vi "Actor Core.vi"(8 "error in":errorcluster, 11 "SensorViewDetailed in":refnum<class "TimerViewDetail.lvclass">) -> (0 "error out":errorcluster, 3 "Actor out":refnum<class "Actor.lvclass">)   [LabVIEW 2012, in "TimerSensor.lvlib" / "TimerViewDetail.lvclass"]
doc: "(<B>Filename</B>: Actor Framework.lvlib:Actor.lvclass:Actor Core.vi)\n\nReceives messages to the actor, reacts to them, and initiates any error handling that may shut the actor down.\n\nDescendant classes may override this VI to append parallel tasks for the actor to complete while it handles messages. Overrides use the Call Parent Method node."
uses:
  TimerViewDetail.lvclass
  <vilib>/ActorFramework/Actor/Actor.lvclass
  Sensor Definition/SensorViewDetailed.lvclass
  <vilib>/ActorFramework/Actor/Actor.lvclass/Actor.ctl
  <vilib>/ActorFramework/Message Enqueuer/Message Enqueuer.lvclass/Message Enqueuer.ctl
  Win8uiFramework/ViewableActor.lvclass/ViewableActor.ctl
  Sensor Definition/SensorView.lvclass/SensorView.ctl
  Sensor Messages/Request Detach Msg/Request Detach Msg.lvclass/Request Detach Msg.ctl
  TimerSensorConfig.lvclass
  Sensor Definition/SensorInfo.lvclass/SensorInfo.ctl
  TimerSensorConfig.lvclass/TimerSensorConfig.ctl
  Sensor Definition/Double Scalar SensorData.lvclass
  Sensor Definition/SensorInfo/Read Description.vi
  Sensor Definition/SensorInfo/Read Name.vi
  Sensor Definition/Read Config.vi
  TimerSensorConfig/Read Target Time.vi
  TimerSensorConfig/Read Timer Direction.vi
  Win8uiFramework/Read Stop Event.vi
  Sensor Definition/SensorView/Read SensorInfo Changed Event.vi
  Sensor Definition/SensorView/Read SensorData Changed Event.vi
  <vilib>/ActorFramework/Message Enqueuer/Init from Existing Queue.vi
  <vilib>/ActorFramework/Message Enqueuer/Enqueue.vi
  <vilib>/ActorFramework/Message Priority Queue/Priority Enqueue.vi
  <vilib>/ActorFramework/Message Enqueuer/Message Enqueuer.lvclass
  Sensor Definition/SensorInfo.lvclass
  Sensor Definition/SensorData.lvclass
  <vilib>/ActorFramework/Stop Msg/Stop Msg.lvclass
  Sensor Messages/Request Display Charm Msg/Request Display Charm Msg.lvclass
  Sensor Messages/Request Detach Msg/Request Detach Msg.lvclass
  Sensor Messages/Shutdown Sensor Msg/Shutdown Sensor Msg.lvclass
  Sensor Definition/SensorConfig.lvclass
  Win8uiFramework/ViewableActor.lvclass
  Win8uiFramework/Win8uiFramework.lvlib
panel:
  out "Title":string="Application Title"
  out "Description":string="Application Title"
  in  "Centered String Hack":bool
  out "Target Time":timestamp format="%<%I:%M:%S %p\n%m/%d/%Y>T"
  in  "Delete":bool
  in  "Open in New Window Button":bool
  in  "Settings":bool
  in  "Back Button":bool
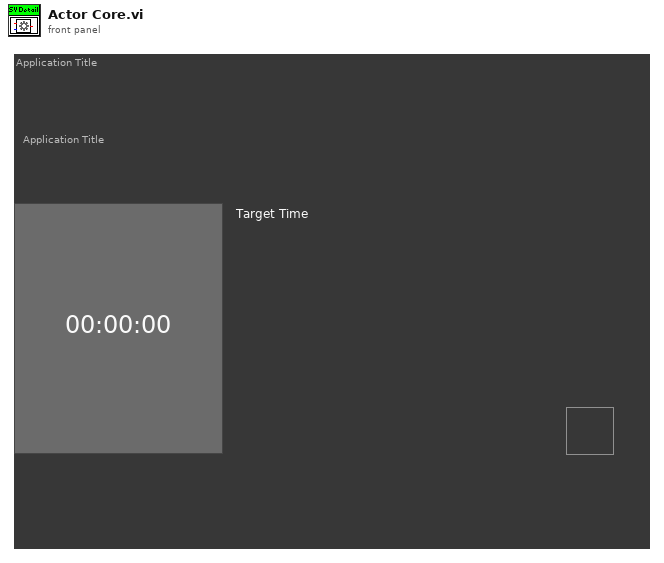
[diagram p1: front panel]
types:
  T1 = typedef "Timer Direction.ctl" = enum16{"Up", "Down"}
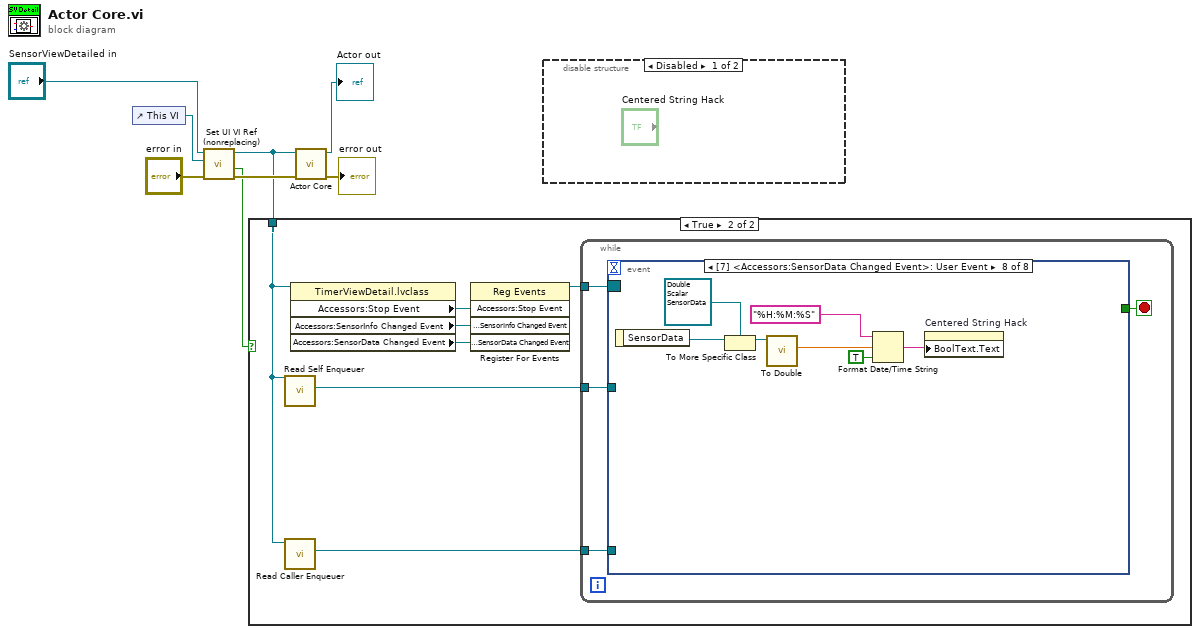
[diagram p0: block diagram]
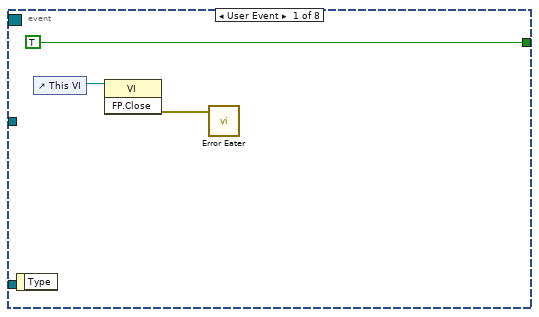
[diagram p4: hidden frame]
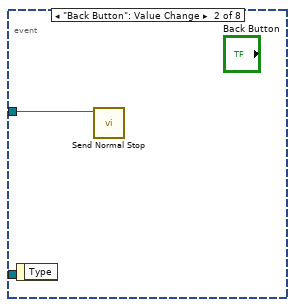
[diagram p5: hidden frame]
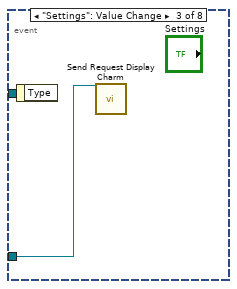
[diagram p6: hidden frame]
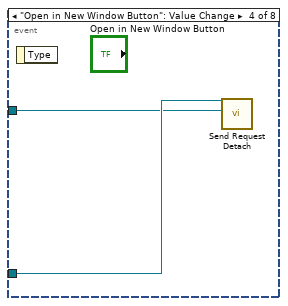
[diagram p7: hidden frame]
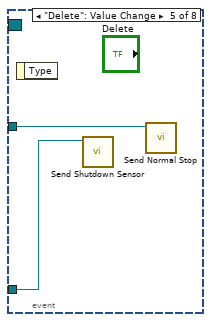
[diagram p8: hidden frame]
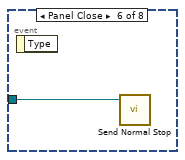
[diagram p9: hidden frame]
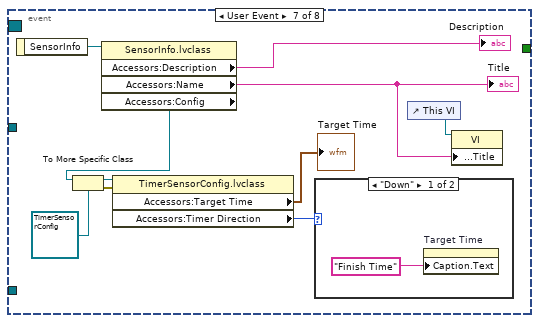
[diagram p10: hidden frame]
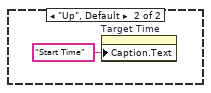
[diagram p11: hidden frame]
diagram:
  n1 = control-ref of="This VI"() -> (w6:refnum<vi>)
  n2 = call "Set UI VI Ref (nonreplacing).vi"("error in (no error)"="error in", "UI VI Ref"=w6, "ViewableActor in"="SensorViewDetailed in") -> ("error out"=w4:errorcluster, "Top Level UI?"=w2:bool, "ViewableActor out"=w3:refnum<class "TimerViewDetail.lvclass">)  [unwired: 6 in]
  n3 = case shown="True" w2 {
    tunnel: w3 -> [_ w10]
    frame False {
    }
    frame True {
      n4 = call <vilib>:"Read Self Enqueuer.vi"("Actor"=w10) -> ("Self Enqueuer"=w11:refnum<class "Message Enqueuer.lvclass">)  [unwired: 10 in]
      n5 = call <vilib>:"Read Caller Enqueuer.vi"("Actor"=w10) -> ("Caller Enqueuer"=w9:refnum<class "Message Enqueuer.lvclass">)  [unwired: 10 in]
      n6 = property class="TimerViewDetail.lvclass"(reference=w10) -> ("Accessors:Stop Event"=w15:refnum<user-event>, "Accessors:SensorInfo Changed Event"=w14:refnum<user-event>, "Accessors:SensorData Changed Event"=w12:refnum<user-event>)  [unwired: 1 in, 2 out]
      n7 = register-events(w15, w14, w12) -> (reference out=w13:refnum<event-registration>)  [unwired: 2 in, 1 out]
      n8 = while {
        tunnel: w13 -> [w19]
        tunnel: w11 -> [w17]
        tunnel: w9 -> [w16]
        stop <- w18 stop-if-true
        n9 = event shown="[7] <Accessors:SensorData Changed Event>: User Event" {
          selector: w19 -> [_ _ _ _ _ _ _ _]
          dyn-events: _ -> [_ _ _ _ _ _ _ _]
          timeout: _ -> [_ _ _ _ _ _ _ _]
          tunnel: [TRUE _ _ _ _ _ _ _] -> w18
          tunnel: w17 -> [_ w23 _ w25 w28 w29 _ _]
          tunnel: w16 -> [_ _ w24 w26 w27 _ _ _]
          event User Event {
            n10 = event-data() -> ()  [unwired: 1 in, 1 out]
            n11 = control-ref of="This VI"() -> (w20:refnum<vi>)
            n12 = invoke class="VI" method="FP.Close"(reference=w20) -> (error out=w21:errorcluster)  [unwired: 2 in, 2 out]
            n13 = call "Error Eater.vi"("error in (no error)"=w21) -> ()  [unwired: 2 in]
          }
          event "Back Button": Value Change {
            n14 = event-data() -> ()  [unwired: 1 in, 1 out]
            n15 = call <vilib>:"Send Normal Stop.vi"("Message Enqueuer"=w23) -> ()  [unwired: 10 in, 1 out]
          }
          event "Settings": Value Change {
            n16 = event-data() -> ()  [unwired: 1 in, 1 out]
            n17 = call "Send Request Display Charm.vi"("Message Enqueuer"=w24) -> ()  [unwired: 9 in, 2 out]
          }
          event "Open in New Window Button": Value Change {
            n18 = event-data() -> ()  [unwired: 1 in, 1 out]
            n19 = call "Send Request Detach.vi"("SensorView Enqueuer"=w25, "Message Enqueuer"=w26) -> ()  [unwired: 8 in, 2 out]
          }
          event "Delete": Value Change {
            n20 = event-data() -> ()  [unwired: 1 in, 1 out]
            n21 = call "Send Shutdown Sensor.vi"("Message Enqueuer"=w27) -> ()  [unwired: 9 in, 2 out]
            n22 = call <vilib>:"Send Normal Stop.vi"("Message Enqueuer"=w28) -> ()  [unwired: 10 in, 1 out]
          }
          event Panel Close {
            n23 = event-data() -> ()  [unwired: 1 in, 1 out]
            n24 = call <vilib>:"Send Normal Stop.vi"("Message Enqueuer"=w29) -> ()  [unwired: 10 in, 1 out]
          }
          event User Event {
            n25 = event-data() -> ("SensorInfo"=w39:refnum<class "SensorInfo.lvclass">)  [unwired: 1 in]
            n26 = property class="SensorInfo.lvclass"(reference=w39) -> ("Accessors:Description"=→"Description":string, "Accessors:Name"=w37:string, "Accessors:Config"=w31:refnum<class "SensorConfig.lvclass">)  [unwired: 1 in, 2 out]
            "Title" <- w37
            n27 = To More Specific Class(target class=refnum<class "TimerSensorConfig.lvclass"> refnum ("TimerSensor.lvlib:TimerSensorConfig.lvclass"), reference=w31) -> (specific class reference=w33:refnum<class "TimerSensorConfig.lvclass">, error out=w34:errorcluster)  [unwired: 1 in]
            n28 = property class="TimerSensorConfig.lvclass"(reference=w33, error in=w34) -> ("Accessors:Target Time"=→"Target Time":timestamp, "Accessors:Timer Direction"=w32:T1)  [unwired: 2 out]
            n29 = case shown="\"Down\"" w32 {
              frame "Down" {
                n30 = property on="Target Time" class="AbsTime (strict)"("Caption.Text"="Finish Time" ("Label.Text")) -> ()  [unwired: 2 in, 2 out]
              }
              frame "Up", Default {
                n31 = property on="Target Time" class="AbsTime (strict)"("Caption.Text"="Start Time" ("Label.Text")) -> ()  [unwired: 2 in, 2 out]
              }
            }
            n32 = control-ref of="This VI"() -> (w38:refnum<vi>)
            n33 = property class="VI"(reference=w38, "Front Panel.Title"=w37) -> ()  [unwired: 1 in, 2 out]
          }
          event User Event {
            n34 = event-data() -> ("SensorData"=w48:refnum<class "SensorData.lvclass">)  [unwired: 1 in]
            n35 = To More Specific Class(target class=refnum<class "Double Scalar SensorData.lvclass"> refnum ("Sensor Definition.lvlib:Double Scalar SensorData.lvclass"), reference=w48) -> (specific class reference=w47:refnum<class "Double Scalar SensorData.lvclass">)  [unwired: 1 in, 1 out]
            n36 = call-dynamic "To Double.vi"("Double Scalar SensorData in"=w47) -> ("Value"=w43:dbl)  [unwired: 8 in, 2 out]
            n37 = Format Date/Time String(time format string (%c)="%H:%M:%S", seconds (now)=w43, UTC format=TRUE) -> (date/time string=w44:string)
            n38 = property on="Centered String Hack" class="Bool (strict)"("BoolText.Text"=w44) -> ()  [unwired: 2 in, 2 out]
          }
        }
      }
    }
  }
  n39 = call-parent "Actor Core.vi"("error in"=w4, "SensorViewDetailed in"=w3) -> ("error out"=→"error out":errorcluster, "Actor out"=→"Actor out":refnum<class "Actor.lvclass">)  [unwired: 8 in]
  n40 = disable-structure shown="Disabled" {
    frame Disabled {
    }
    frame Enabled {
    }
  }
